vi "test_MonoAllTests.vi"(6 "init mono?":bool, 7 "Test should pass":bool=TRUE, 8 "error in":errorcluster, 9 "tear down connection":bool=TRUE, 10 "set-up a connection":bool=TRUE, 11 "device selection":enum16{"monochromator", "CCD", "SCD"}(ring)) -> (0 "error out":errorcluster, 1 "log-file path":path)   [LabVIEW 2023]
uses:
  Classes/CCD/CCD.lvclass
  C:/Projects/Horiba/horiba-labview-sdk/Source/Classes/GenericDevice/GenericDevice.lvclass
  <vilib>/addons/_JKI Toolkits/Caraya/classes/Test/Test.lvclass
  <vilib>/Hampel Software Engineering/HSE Logger/hse-logger.lvlib
panel:
  # "Connector Pane"
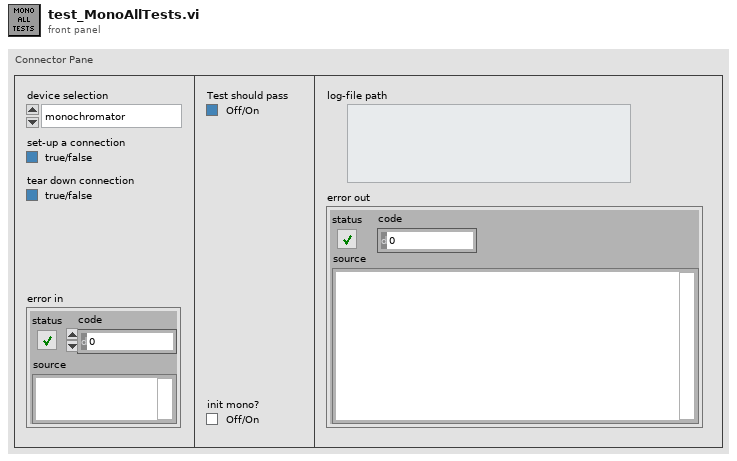
[diagram p1: front panel]
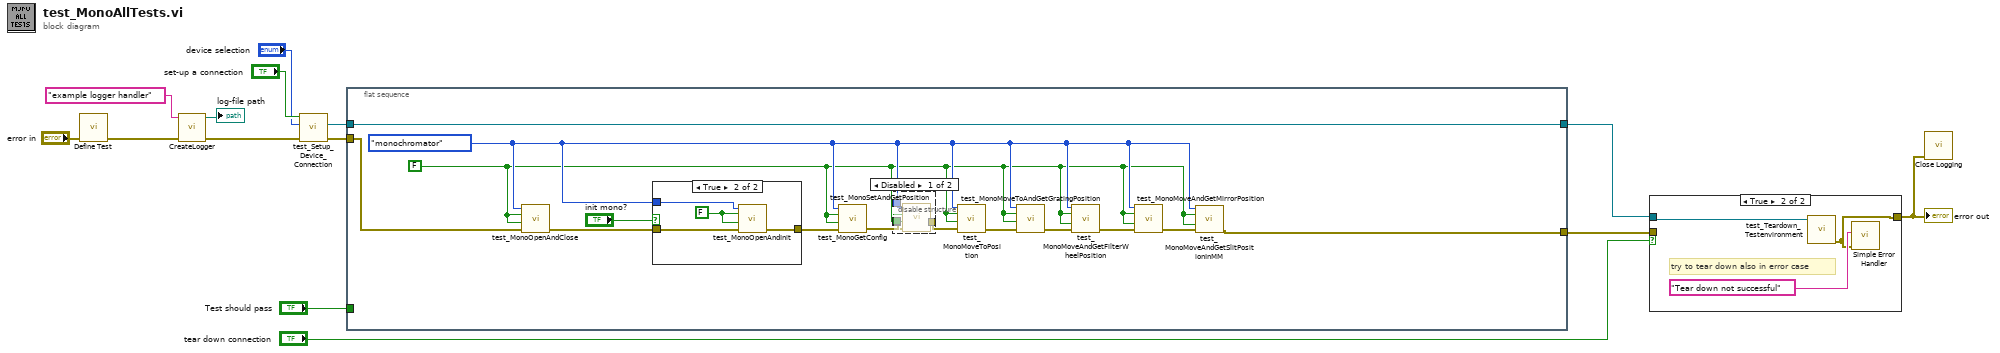
[diagram p0: block diagram]
diagram:
  n1 = call <vilib>:"Define Test.vi"("error in (no error)"="error in") -> ("error out"=w4:errorcluster)  [unwired: 9 in, 1 out]
  n2 = call "CreateLogger.vi"("error in (no error)"=w4, "Handler Name"="example logger handler") -> ("error out"=w3:errorcluster, "log-file path"=→"log-file path":path)  [unwired: 8 in]
  n3 = call "test_Setup_Device_Connection.vi"("error in (no error)"=w3, "device selection"="device selection", "set-up a connection"="set-up a connection") -> ("error out"=w7:errorcluster, "CCD.lvclass"=w8:refnum<class "CCD.lvclass">)  [unwired: 5 in, 2 out]
  n4 = flat-sequence {
    tunnel: w7 -> [w27]
    tunnel: w8 -> [w28]
    tunnel: "Test should pass" -> [_]
    tunnel: [w28] -> w11
    tunnel: [w17] -> w1
    frame #0 {
      w20 = enum16{"monochromator", "CCD", "SCD"}."monochromator" ("device selection")
      w19 = FALSE
      n5 = call "test_MonoOpenAndClose.vi"("error in"=w27, "tear down connection"=w19, "set-up a connection"=w19, "device selection"=w20) -> ("error out"=w25:errorcluster)  [unwired: 6 in, 1 out]
      n6 = case shown="True" "init mono?" {
        tunnel: w25 -> [w33 w37]
        tunnel: w20 -> [_ w35]
        tunnel: [w33 w34] -> w24
        frame False {
        }
        frame True {
          w36 = FALSE
          n7 = call "test_MonoOpenAndInit.vi"("error in"=w37, "tear down connection"=w36, "set-up a connection"=w36, "device selection"=w35) -> ("error out"=w34:errorcluster)  [unwired: 6 in, 1 out]
        }
      }
      n8 = call "test_MonoGetConfig.vi"("error in"=w24, "tear down connection"=w19, "set-up a connection"=w19, "device selection"=w20) -> ("error out"=w23:errorcluster)  [unwired: 6 in, 1 out]
      n9 = disable-structure shown="Disabled" {
        disable-tunnel: w23 -> [w32 _]
        disable-tunnel: [w31 _] -> w22
        disable-tunnel: w20 -> [w30 _]
        disable-tunnel: w19 -> [w29 _]
        frame Disabled {
          n10 = call "test_MonoSetAndGetPosition.vi"("error in"=w32, "tear down connection"=w29, "set-up a connection"=w29, "device selection"=w30) -> ("error out"=w31:errorcluster)  [unwired: 6 in, 1 out]
        }
        frame Enabled {
        }
      }
      n11 = call "test_MonoMoveToPosition.vi"("device selection"=w20, "set-up a connection"=w19, "tear down connection"=w19, "error in"=w22) -> ("error out"=w16:errorcluster)  [unwired: 7 in, 4 out]
      n12 = call "test_MonoMoveToAndGetGratingPosition.vi"("device selection"=w20, "set-up a connection"=w19, "tear down connection"=w19, "error in"=w16) -> ("error out"=w21:errorcluster)  [unwired: 7 in, 4 out]
      n13 = call "test_MonoMoveAndGetFilterWheelPosition.vi"("device selection"=w20, "set-up a connection"=w19, "tear down connection"=w19, "error in"=w21) -> ("error out"=w15:errorcluster)  [unwired: 10 in, 1 out]
      n14 = call "test_MonoMoveAndGetMirrorPosition.vi"("device selection"=w20, "set-up a connection"=w19, "tear down connection"=w19, "error in"=w15) -> ("error out"=w18:errorcluster)  [unwired: 7 in, 4 out]
      n15 = call "test_MonoMoveAndGetSlitPositionInMM.vi"("device selection"=w20, "set-up a connection"=w19, "tear down connection"=w19, "error in"=w18) -> ("error out"=w17:errorcluster)  [unwired: 10 in, 1 out]
    }
  }
  n16 = case shown="True" "tear down connection" {
    tunnel: w11 -> [_ w40]
    tunnel: [w38 w39] -> w2
    tunnel: w1 -> [w38 _]
    frame False {
    }
    frame True {
      # "try to tear down also in error case"
      n17 = call "test_Teardown_Testenvironment.vi"("GenericDevice.lvclass"=w40) -> ("error out"=w39:errorcluster)  [unwired: 9 in, 1 out]
      n18 = call <vilib>:"Simple Error Handler.vi"("error source (\" \")"="Tear down not successful" ("error source (\" \")"), "error in (no error)"=w39) -> ()  [unwired: 3 in, 5 out]
    }
  }
  "error out" <- w2
  n19 = call <vilib>:"Close Logging.vi"("error in"=w2) -> ()  [unwired: 10 in, 1 out]
